vi "stitch.vi"(6 "offsets":dbl[](array[numeric]), 7 "f(x,a)":T1, 8 "splice params":dbl[][](array[numeric]), 9 "a":dbl[][](array[numeric]), 10 "splice count":i32, 11 "X":dbl[](array[numeric])) -> (2 "f(X, a)":dbl[](array[numeric]))   [LabVIEW 2019]
uses:
  <vilib>/gmath/NumericalOptimization/LM model function reference.ctl
  <vilib>/gmath/NI_Gmath.lvlib
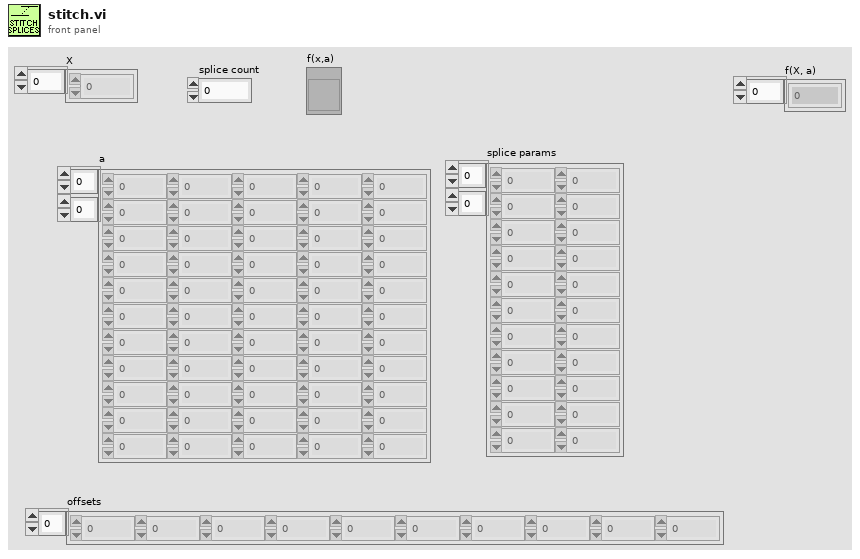
[diagram p1: front panel]
types:
  T1 = typedef "NI_Gmath.lvlib/LM model function reference.ctl" = refnum<vi>
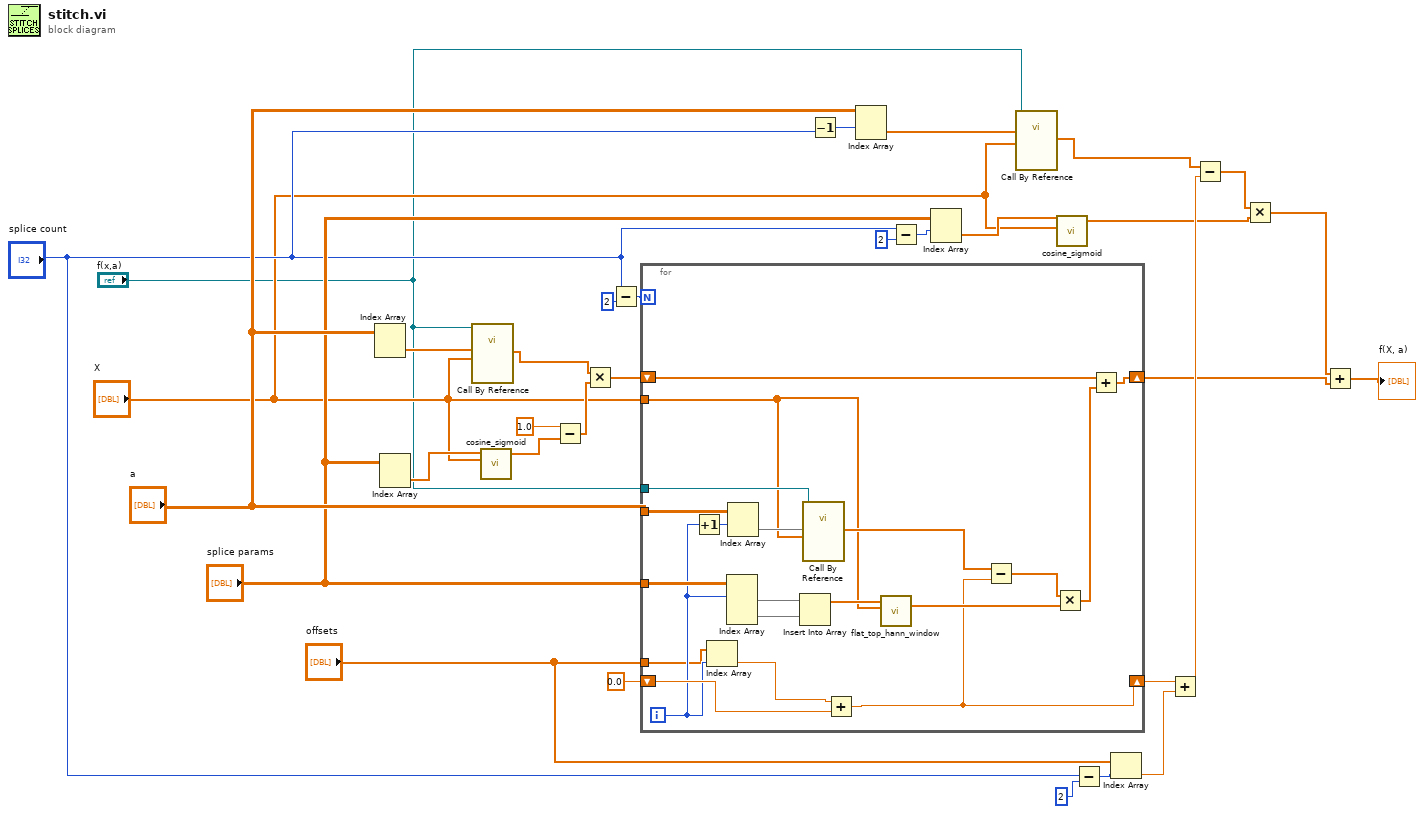
[diagram p0: block diagram]
diagram:
  n1 = Index Array(array="a") -> (element=w10:dbl[])  [unwired: 2 in]
  n2 = Index Array(array="splice params") -> (element=w7:dbl[])  [unwired: 2 in]
  n3 = call-by-ref "?"(reference="f(x,a)", "X"="X", "a"=w10) -> ("f(X,a)"=w9:dbl[])  [unwired: 3 in, 4 out]
  n4 = call "cosine_sigmoid.vi"("X"="X", "a"=w7) -> ("f(X,a)"=w8:dbl[])  [unwired: 2 in, 2 out]
  n5 = Subtract(x=1.0, y=w8) -> (x-y=w28:dbl[])
  n6 = Multiply(x=w9, y=w28) -> (x*y=w27:dbl[])
  n7 = Subtract(x="splice count", y=2) -> (x-y=w30:i32)
  n8 = for {
    N: w30 -> [_]
    shift-right: [w37] -> w21
    shift-left: 0.0 -> [w36]
    tunnel: "offsets" -> [w34]
    tunnel: "X" -> [w38]
    tunnel: "a" -> [w50]
    tunnel: "splice params" -> [w52]
    shift-right: [w48] -> w12
    shift-left: w27 -> [w47]
    tunnel: "f(x,a)" -> [w43]
    i -> [w35]
    n9 = Increment(x=w35) -> (x+1=w51:i32)
    n10 = Index Array(array=w34, index=w35) -> (element=w33:dbl)
    n11 = Index Array(array=w52, index (row) #1=w35) -> (element #1=w41:dbl[], element #2=w40:dbl[])  [unwired: 3 in]
    n12 = Index Array(array=w50, index (row)=w51) -> (element=w44:dbl[])  [unwired: 1 in]
    n13 = Insert Into Array(array=w41, new element=w40) -> (w39:dbl[])  [unwired: 1 in]
    n14 = call-by-ref "?"(reference=w43, "X"=w38, "a"=w44) -> ("f(X,a)"=w45:dbl[])  [unwired: 3 in, 4 out]
    n15 = Add(x=w33, y=w36) -> (x+y=w37:dbl)
    n16 = call "flat_top_hann_window.vi"("X"=w38, "a"=w39) -> ("f(X,a)"=w42:dbl[])  [unwired: 2 in, 2 out]
    n17 = Subtract(x=w45, y=w37) -> (x-y=w49:dbl[])
    n18 = Multiply(x=w49, y=w42) -> (x*y=w46:dbl[])
    n19 = Add(x=w47, y=w46) -> (x+y=w48:dbl[])
  }
  n20 = Decrement(x="splice count") -> (x-1=w26:i32)
  n21 = Index Array(array="a", index (row)=w26) -> (element=w4:dbl[])  [unwired: 1 in]
  n22 = Subtract(x="splice count", y=2) -> (x-y=w23:i32)
  n23 = Index Array(array="splice params", index (row)=w23) -> (element=w6:dbl[])  [unwired: 1 in]
  n24 = call-by-ref "?"(reference="f(x,a)", "X"="X", "a"=w4) -> ("f(X,a)"=w2:dbl[])  [unwired: 3 in, 4 out]
  n25 = call "cosine_sigmoid.vi"("X"="X", "a"=w6) -> ("f(X,a)"=w5:dbl[])  [unwired: 2 in, 2 out]
  n26 = Subtract(x="splice count", y=2) -> (x-y=w18:i32)
  n27 = Index Array(array="offsets", index=w18) -> (element=w16:dbl)
  n28 = Add(x=w21, y=w16) -> (x+y=w15:dbl)
  n29 = Subtract(x=w2, y=w15) -> (x-y=w14:dbl[])
  n30 = Multiply(x=w14, y=w5) -> (x*y=w13:dbl[])
  n31 = Add(x=w13, y=w12) -> (x+y=→"f(X, a)":dbl[])
